vi "load_class.vi"(7 "config in":T1, 8 "error in (no error)":errorcluster, 11 "lv-builder in":refnum<class "lv-builder.lvclass">) -> (0 "error out":errorcluster, 3 "lv-builder out":refnum<class "lv-builder.lvclass">)   [LabVIEW 2015, in "lv-build-interface.lvlib"]
uses:
  lv-build-interface.lvlib
  lv-builder/class/lv-builder.lvclass
  lv-build/public/_controls/configuration.ctl
  lv-builder/lv-builder.lvlib
  lv-build/lv-build.lvlib
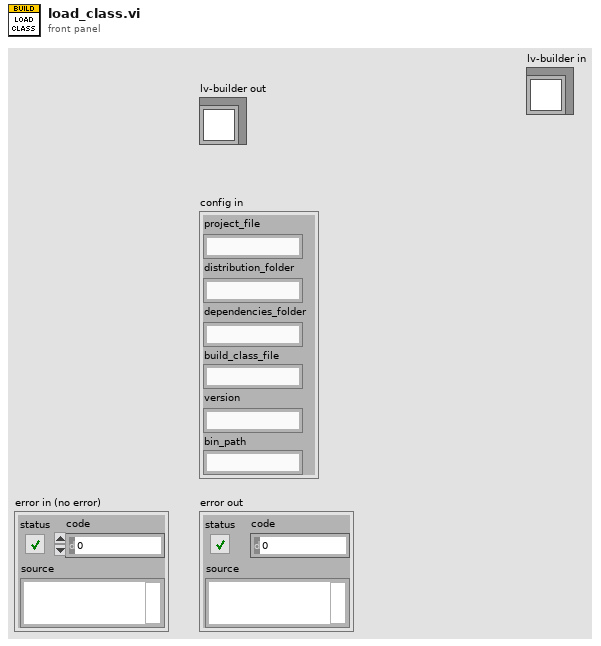
[diagram p1: front panel]
types:
  T1 = typedef "lv-build.lvlib/configuration.ctl" = cluster{"project_file":string, "distribution_folder":string, "dependencies_folder":string, "build_class_file":string, "version":string, "bin_path":string}
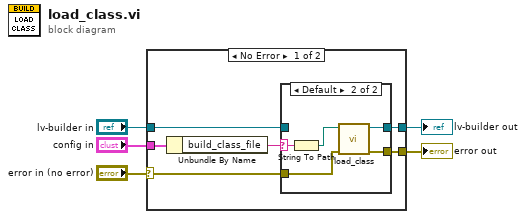
[diagram p0: block diagram]
diagram:
  n1 = case shown="No Error" "error in (no error)" {
    selector: "error in (no error)" -> [w10 w20]
    tunnel: "config in" -> [w11 _]
    tunnel: [w9 w20] -> w4
    tunnel: "lv-builder in" -> [w8 w19]
    tunnel: [w7 w19] -> w2
    frame No Error {
      n2 = Unbundle By Name(w11) -> ("build_class_file"=w6:string)
      n3 = case shown="Default" w6 {
        selector: w6 -> [_ w18]
        tunnel: w10 -> [w13 w16]
        tunnel: [w13 w15] -> w9
        tunnel: w8 -> [w12 _]
        tunnel: [w12 w14] -> w7
        frame "" {
        }
        frame Default {
          n4 = String To Path(string=w18) -> (path=w17:path)
          n5 = call "load_class.vi"("error in (no error)"=w16, "class"=w17) -> ("error out"=w15:errorcluster, "lv_build_plugin"=w14:refnum<class "lv-builder.lvclass">)  [unwired: 8 in]
        }
      }
    }
    frame Error {
    }
  }
  "lv-builder out" <- w2
  "error out" <- w4
